vi "Read-Write Vision Settings to File.vi"(6 "Read(f)Write(t)":bool, 7 "Target":T3, 8 "Error":errorcluster, 11 "Vision Settings":T1={"Color"={"Hue"={235.0, 13.0}, "Sat"={97.0, 224.64285714285714}, "Val"={170.0, 255.0}}, "Particles"=10.0, "Score Cutoff"=50.0, "Line Border"={"Top"=6.0, "Bottom"=1.0}, "Size Limit %"=0.04} {"Color"."Hue" scale=0.0..255.0 scale format="%#_3g"}) -> (0 "Error Out":errorcluster, 3 "Vision Settings Out":T1={"Color"={"Hue"={235.0, 13.0}, "Sat"={97.0, 224.64285714285714}, "Val"={170.0, 255.0}}, "Particles"=10.0, "Score Cutoff"=50.0, "Line Border"={"Top"=6.0, "Bottom"=1.0}, "Size Limit %"=0.04} {"Color"."Hue" scale=0.0..255.0 scale format="%#_3g"}, 5 "Found? Out":bool)   [LabVIEW 2017, in "VisionSystem.lvlib"]
uses:
  VisionSystem.lvlib
  Enum_ Field Targets.ctl
  Cluster_Vision Settings.ctl
  Cluster_Threshold Settings.ctl
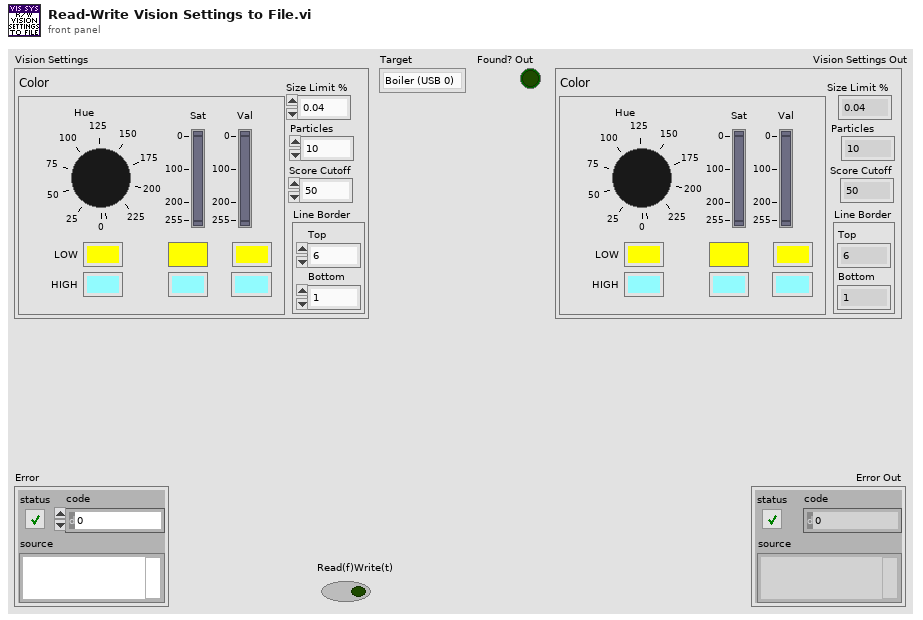
[diagram p1: front panel]
types:
  T1 = typedef "VisionSystem.lvlib/Cluster_Vision Settings.ctl" = cluster{"Color":T2, "Particles":dbl, "Score Cutoff":dbl, "Line Border":cluster{"Top":dbl, "Bottom":dbl}, "Size Limit %":dbl}
  T2 = typedef "VisionSystem.lvlib/Cluster_Threshold Settings.ctl" = cluster{"Hue":cluster{dbl, dbl}, "Sat":cluster{dbl, dbl}, "Val":cluster{dbl, dbl}}
  T3 = typedef "VisionSystem.lvlib/Enum_ Field Targets.ctl" = enum16{"Boiler (USB 0)", "Rope (USB 1)"}
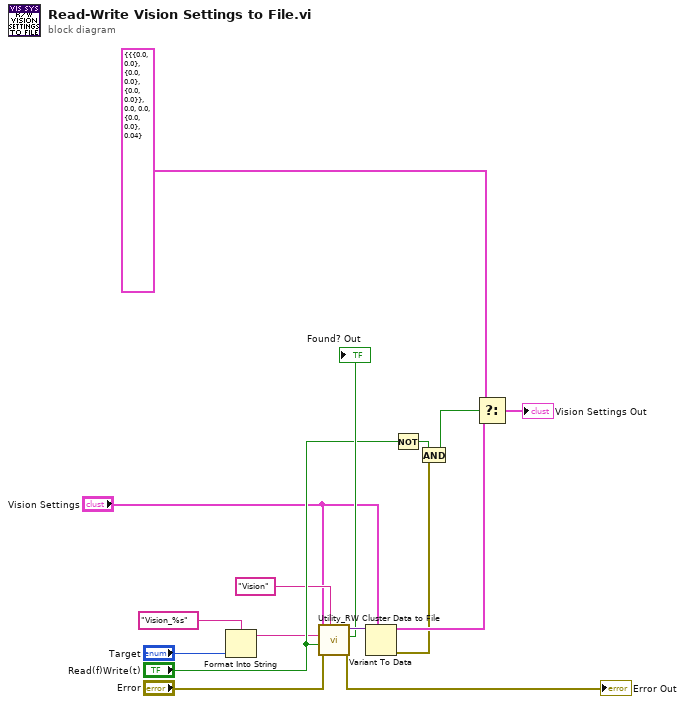
[diagram p0: block diagram]
diagram:
  n1 = Format Into String(format string="Vision_%s", "Target") -> (resulting string=w6:string)  [unwired: 2 in, 1 out]
  n2 = call "Utility_RW Cluster Data to File.vi"("System"="Vision" ("File Name"), "Error"="Error", "Read(f)Write(t)"="Read(f)Write(t)", "Data Name"=w6, "Cluster Data"="Vision Settings") -> ("Error Out"=→"Error Out":errorcluster, "Found? Out"=→"Found? Out":bool, "Cluster Data Out"=w13:variant)  [unwired: 4 in]
  n3 = Variant To Data(type="Vision Settings", Variant=w13) -> (data=w12:T1, error out=w7:errorcluster)  [unwired: 1 in]
  n4 = Not(x="Read(f)Write(t)") -> (.not. x?=w9:bool)
  n5 = And(x=w9, y=w7) -> (x .and. y?=w8:bool)
  n6 = Select(t=T1 {"Color"={"Hue"={0.0, 0.0}, "Sat"={0.0, 0.0}, "Val"={0.0, 0.0}}, "Particles"=0.0, "Score Cutoff"=0.0, "Line Border"={"Top"=0.0, "Bottom"=0.0}, "Size Limit %"=0.04} ("Vision Settings"), s=w8, f=w12) -> (s? t:f=→"Vision Settings Out":T1)
